vi "CONVnano.vi"(9 "vAL":dbl) -> (1 "NANO":dbl)   [LabVIEW 2018]
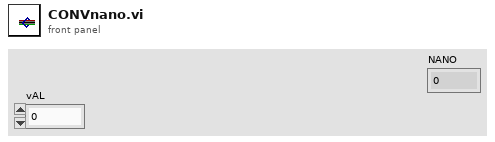
[diagram p1: front panel]
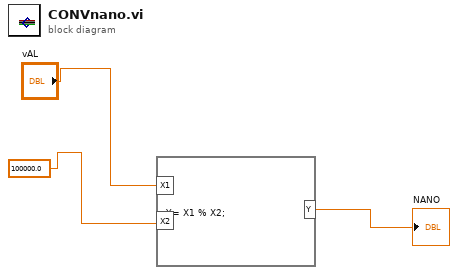
[diagram p0: block diagram]
diagram:
  n1 = formula code="Y= X1 % X2;"("X1"="vAL", "X2"=100000.0 ("y")) -> ("Y"=→"NANO":dbl)
